vi "TestCreateNewDirectory.vi"(1 "NewDirectory":string) -> (0 "NewDirectoryReturn":string)   [LabVIEW 2021]
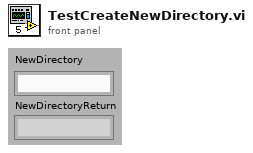
[diagram p1: front panel]
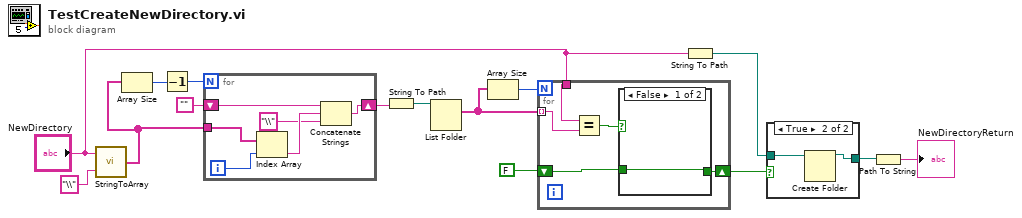
[diagram p0: block diagram]
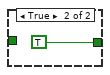
[diagram p3: hidden frame]
diagram:
  n1 = call "StringToArray.vi"("String Delimiter"="\\", "Input String"="NewDirectory") -> ("Array"=w3:string[])
  n2 = Array Size(array=w3) -> (size(s)=w13:i32)
  n3 = Decrement(x=w13) -> (x-1=w14:i32)
  n4 = for {
    N: w14 -> [_]
    tunnel: w3 -> [w20]
    shift-right: [w16] -> w11
    shift-left: "" -> [w19]
    i -> [w21]
    n5 = Index Array(array=w20, index=w21) -> (element=w18:string)
    n6 = Concatenate Strings(w19, w18, "\\") -> (w16:string)
  }
  n7 = String To Path(string=w11) -> (path=w10:path)
  n8 = List Folder(path=w10) -> (filenames=w8:string[])  [unwired: 3 in, 3 out]
  n9 = Array Size(array=w8) -> (size(s)=w9:i32)
  n10 = for {
    N: w9 -> [_]
    tunnel: w8 -> [w25] mode=indexing
    tunnel: "NewDirectory" -> [w26]
    shift-right: [w22] -> w6
    shift-left: FALSE -> [w23]
    n11 = Equal?(x=w26, y=w25) -> (x = y?=w24:bool)
    n12 = case shown="False" w24 {
      tunnel: w23 -> [w27 _]
      tunnel: [w27 TRUE] -> w22
      frame False {
      }
      frame True {
      }
    }
  }
  n13 = String To Path(string="NewDirectory") -> (path=w4:path)
  n14 = case shown="True" w6 {
    tunnel: w4 -> [w29 w31]
    tunnel: [w29 w30] -> w2
    frame False {
    }
    frame True {
      n15 = Create Folder(path (use dialog)=w31) -> (created path=w30:path)  [unwired: 2 in, 2 out]
    }
  }
  n16 = Path To String(path=w2) -> (string=→"NewDirectoryReturn":string)
